vi "Scripting_GetTerminalWireConnectionPoints.vi"(0 "Term Refnum In":refnum<vi>, 1 "ControlRef(IgnoredIfNotWired)":refnum<vi>, 5 "error in":errorcluster, 8 "RemoveWire(False)":bool) -> (11 "Data Type":variant, 12 "IsTheSource":bool, 13 "AllWireTerminals":refnum<vi>[](array[refnum]), 14 "Term Refnum Out":refnum<vi>, 15 "WireTermSource":refnum<vi>, 16 "FirstWireTermDrain":refnum<vi>, 17 "NoWireConnected":bool, 18 "AllWireTerminalDrains":refnum<vi>[](array[refnum]), 19 "error out":errorcluster)   [LabVIEW 2020]
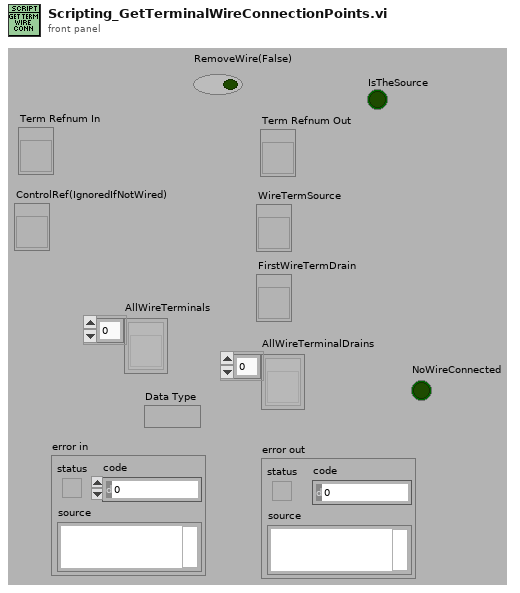
[diagram p1: front panel]
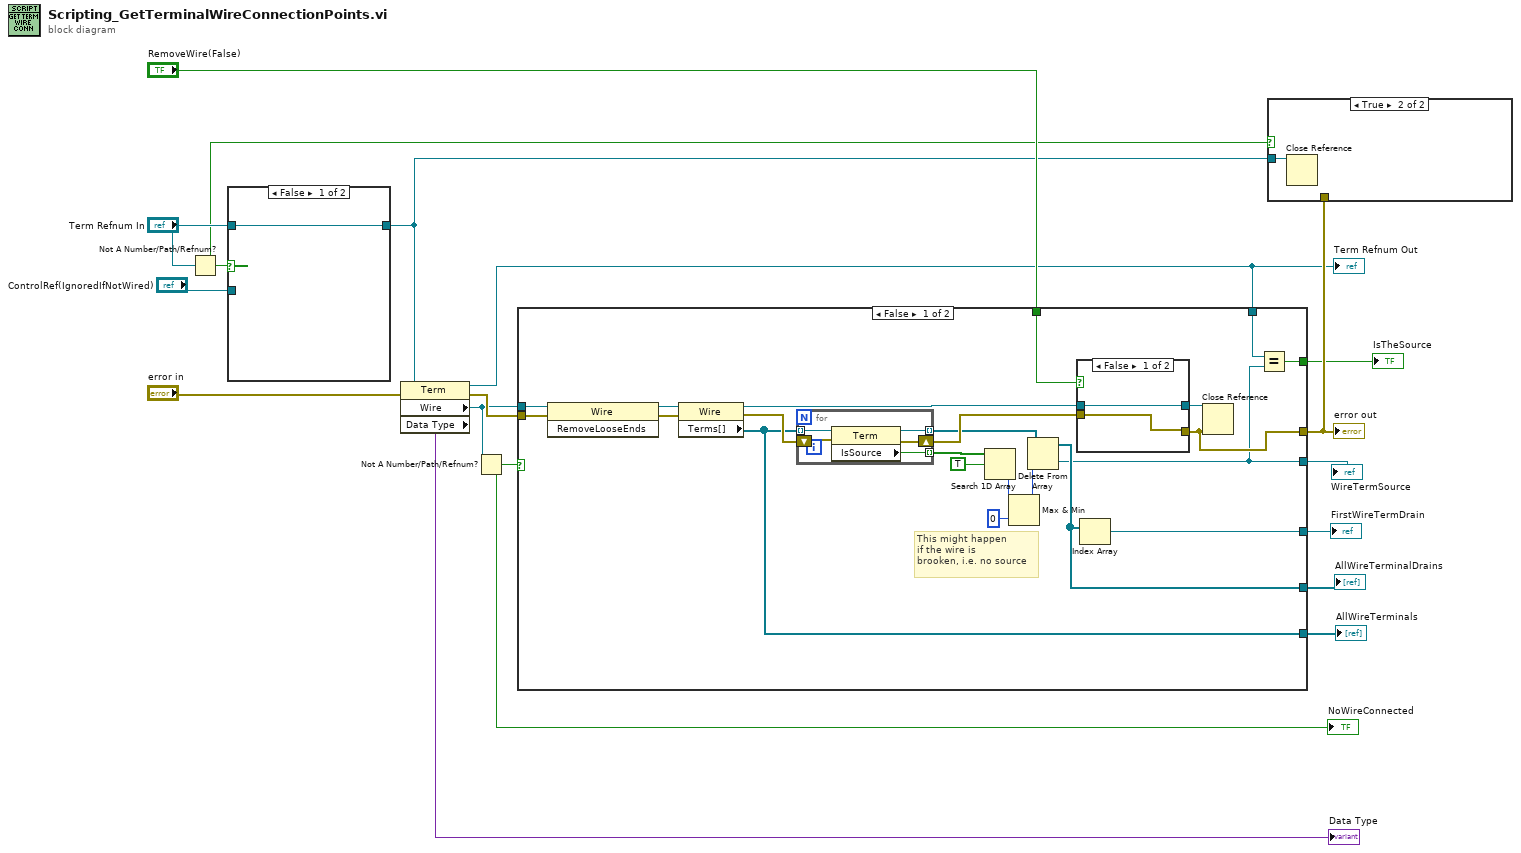
[diagram p0: block diagram]
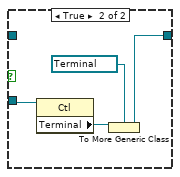
[diagram p3: hidden frame]
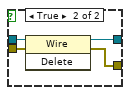
[diagram p4: hidden frame]
diagram:
  n1 = Not A Number/Path/Refnum?(number/path/refnum="Term Refnum In") -> (NaN/Path/Refnum?=w5:bool)
  n2 = case shown="False" w5 {
    tunnel: "Term Refnum In" -> [w18 _]
    tunnel: [w18 w19] -> w4
    tunnel: "ControlRef(IgnoredIfNotWired)" -> [_ w22]
    frame False {
    }
    frame True {
      n3 = property class="Ctl"(reference=w22) -> ("Terminal"=w21:refnum<vi>)  [unwired: 1 in, 2 out]
      n4 = To More Generic Class(target class=refnum<vi> refnum ("Term Refnum In"), reference=w21) -> (generic class reference=w19:refnum<vi>)
    }
  }
  n5 = property class="Term"(reference=w4, error in="error in") -> (reference out=w3:refnum<vi>, error out=w16:errorcluster, "Wire"=w10:refnum<vi>, "Data Type"=→"Data Type":variant)
  "Term Refnum Out" <- w3
  n6 = Not A Number/Path/Refnum?(number/path/refnum=w10) -> (NaN/Path/Refnum?=w9:bool)
  "NoWireConnected" <- w9
  n7 = case shown="False" w9 {
    tunnel: w16 -> [w25 w56]
    tunnel: "RemoveWire(False)" -> [w37 _]
    tunnel: [w28 _] -> w14
    tunnel: [w36 _] -> w13
    tunnel: [w35 _] -> w12
    tunnel: [w34 _] -> w11
    tunnel: [w33 w56] -> w6
    tunnel: w10 -> [w26 _]
    tunnel: w3 -> [w29 _]
    tunnel: [w27 _] -> w2
    frame False {
      # "This might happen\nif the wire is\nbrooken, i.e. no source"
      n8 = invoke class="Wire" method="RemoveLooseEnds"(reference=w26, error in=w25) -> (reference out=w24:refnum<vi>, error out=w23:errorcluster)  [unwired: 1 in, 1 out]
      n9 = property class="Wire"(reference=w24, error in=w23) -> (reference out=w42:refnum<vi>, error out=w41:errorcluster, "Terms[]"=w34:refnum<vi>[])
      n10 = for {
        tunnel: w34 -> [w55] mode=indexing
        tunnel: [w54] -> w38 mode=indexing
        tunnel: [w53] -> w40 mode=indexing
        shift-right: [w51] -> w43
        shift-left: w41 -> [w52]
        n11 = property class="Term"(reference=w55, error in=w52) -> (reference out=w53:refnum<vi>, error out=w51:errorcluster, "IsSource"=w54:bool)
      }
      n12 = Search 1D Array(1D array=w38, element=TRUE) -> (index of element=w31:i32)  [unwired: 1 in]
      n13 = Max & Min(x=w31, y=0) -> (max(x,y)=w30:i32)  [unwired: 1 out]
      n14 = Delete From Array(array=w40, index=w30) -> (deleted portion=w28:refnum<vi>, array with subset deleted=w36:refnum<vi>[])  [unwired: 1 in]
      n15 = case shown="False" w37 {
        tunnel: [w45 w50] -> w33
        tunnel: [w46 w49] -> w44
        tunnel: w43 -> [w45 w48]
        tunnel: w42 -> [w46 w47]
        frame False {
        }
        frame True {
          n16 = invoke class="Wire" method="Delete"(reference=w47, error in=w48) -> (reference out=w49:refnum<vi>, error out=w50:errorcluster)  [unwired: 1 in, 1 out]
        }
      }
      n17 = Index Array(array=w36) -> (element=w35:refnum<vi>)  [unwired: 1 in]
      n18 = Close Reference(reference=w44, error in (no error)=w33) -> ()  [unwired: 1 out]
      n19 = Equal?(x=w29, y=w28) -> (x = y?=w27:bool)
    }
    frame True {
    }
  }
  "error out" <- w6
  "WireTermSource" <- w14
  "FirstWireTermDrain" <- w12
  "AllWireTerminalDrains" <- w13
  "AllWireTerminals" <- w11
  "IsTheSource" <- w2
  n20 = case shown="True" w5 {
    tunnel: w6 -> [_ _]
    tunnel: w4 -> [_ w57]
    frame False {
    }
    frame True {
      n21 = Close Reference(reference=w57) -> ()  [unwired: 1 in, 1 out]
    }
  }
